vi "update.vi"(8 "error in (no error)":errorcluster, 10 "Model in":refnum<class "Model.lvclass">, 11 "EnabledState in":refnum<class "EnabledState.lvclass">) -> (0 "error out":errorcluster, 2 "Model out":refnum<class "Model.lvclass">, 3 "EnabledState out":refnum<class "EnabledState.lvclass">)   [LabVIEW 2015, in "EnabledState.lvclass"]
uses:
  EnabledState.lvclass
  Model/Model/Model.lvclass
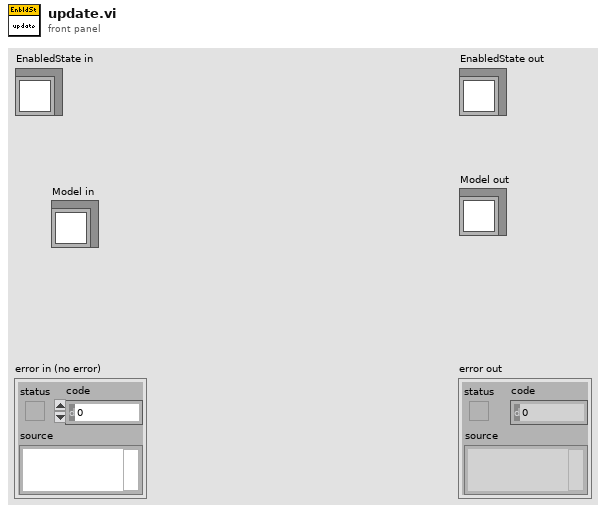
[diagram p1: front panel]
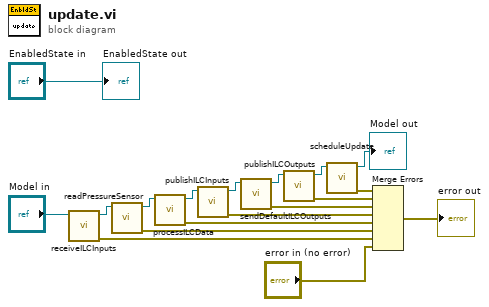
[diagram p0: block diagram]
diagram:
  n1 = call "receiveILCInputs.vi"("Model in"="Model in") -> ("error out"=w13:errorcluster, "Model out"=w3:refnum<class "Model.lvclass">)  [unwired: 9 in]
  n2 = call "readPressureSensor.vi"("Model in"=w3) -> ("error out"=w1:errorcluster, "Model out"=w2:refnum<class "Model.lvclass">)  [unwired: 9 in]
  n3 = call "processILCData.vi"("Model in"=w2) -> ("error out"=w12:errorcluster, "Model out"=w9:refnum<class "Model.lvclass">)  [unwired: 9 in]
  n4 = call "publishILCInputs.vi"("Model in"=w9) -> ("error out"=w7:errorcluster, "Model out"=w8:refnum<class "Model.lvclass">)  [unwired: 9 in]
  n5 = call "sendDefaultILCOutputs.vi"("Model in"=w8) -> ("error out"=w10:errorcluster, "Model out"=w6:refnum<class "Model.lvclass">)  [unwired: 9 in]
  n6 = call "publishILCOutputs.vi"("Model in"=w6) -> ("error out"=w4:errorcluster, "Model out"=w5:refnum<class "Model.lvclass">)  [unwired: 9 in]
  n7 = call "scheduleUpdate.vi"("Model in"=w5) -> ("error out"=w11:errorcluster, "Model out"=→"Model out":refnum<class "Model.lvclass">)  [unwired: 9 in]
  n8 = Merge Errors(w11, w4, w10, w7, w12, w1, w13, "error in (no error)") -> (→"error out":errorcluster)
  "EnabledState out" <- "EnabledState in"
